vi "test - #98.vi"(8 "error in (no error)":errorcluster, 11 "TestCase in":refnum<class "testcase-Supported-Datatype.lvclass">) -> (0 "error out":errorcluster, 3 "TestCase out":refnum<class "testcase-Supported-Datatype.lvclass">)   [LabVIEW 2017, in "testcase-Supported-Datatype.lvclass"]
uses:
  testcase-Supported-Datatype.lvclass
  fb94dfaf-6f85-427f-a0fa-1e7f335e48cb.vi
  e57ab7a4-7139-4cc0-9c10-fbc2ee1cf7e2.vi
  addons/API-String-Arugments-Support/_Support/Data To API String Arguments.vi
  addons/API-String-Arugments-Support/_Support/Convert API String Arguments to Data(variant).vi
  <vilib>/addons/_JKI Toolkits/VI Tester/TestCase.llb/TestCase.lvclass
  C:/Program Files (x86)/National Instruments/LabVIEW 2017/vi.lib/addons/_JKI Toolkits/VI Tester/TestCase.llb/TestCase.lvclass
panel:
  out "String 2":string
  out "Stimulus 3":T1={"Stimulus Type"=enum."Frequency Stepped Sweep", "Custom Stimulus Name"="", "Apply EQ"=FALSE, "Advanced View"=FALSE, "Sampling Rate"="Device Default", "Output Path"={"Output Path"="", "Sampling Rate"=48000}, "Frequency Stepped Sweep"={"Level"=0.35, "Unit"=0, "Resolution"=1, "Start (Hz)"=10000.0, "Stop (Hz)"=100.0, "Min cycles (#)"=10.0, "Min Duration (s)"=0.01, "Steps (#)"=0}, "Frequency Log Sweep"={"Level"=0.35, "Unit"=0, "Start (Hz)"=100.0, "Stop (Hz)"=10000.0, "Sweep Time (s)"=2.0}, "Log Amplitude Sweep"={"Freq"=1000.0, "Steps (#)"=20.0, "Start"=1.0, "Unit"=0, "Cycles （#)"=10.0, "Stop"=2.0}, "WAV"={"Level"=0.35, "Unit"=0, "WAV File Path"=path "", "WAV File Channel"=0}, "Noise"={"Level"=0.35, "Unit"=0, "Noise Type"=enum."Pink Noise", "Min (Hz)"=100.0, "Max (Hz)"=20000.0, "Duration (s)"=2.0}, "Multitone"={"Level"=0.35, "Unit"=0, "Resolution"=1, "Min (Hz)"=100.0, "Max (Hz)"=10000.0, "Duration (s)"=2.0, "Tones (#)"=10}, "Stimulus List"=[]} {"Multitone"."Duration (s)" format="%#_6p"; "Multitone"."Max (Hz)" format="%#_6p"; "Multitone"."Min (Hz)" format="%#_6p"; "Multitone"."Resolution" items=["R10 (1/3 Oct.)", "R20 (1/6 Oct.)", "R40 (1/12 Oct.)", "R80 (1/24 Oct.)", "User Def. Log", "User Def. Lin"]; "Multitone"."Unit" items=["V RMS"]; "Multitone"."Level" format="%#_6p"; "Noise"."Max (Hz)" format="%#_6p"; "Noise"."Min (Hz)" format="%#_6p"; "Noise"."Unit" items=["V RMS"]; "Noise"."Level" format="%#_6p"; "WAV"."WAV File Channel" items=["Mono"]; "WAV"."Unit" items=["V RMS"]; "WAV"."Level" format="%#_6p"; "Log Amplitude Sweep"."Stop" format="%#_6p"; "Log Amplitude Sweep"."Cycles （#)" format="%#_6p"; "Log Amplitude Sweep"."Unit" items=["V RMS"]; "Log Amplitude Sweep"."Start" format="%#_6p"; "Log Amplitude Sweep"."Steps (#)" format="%#_6p"; "Log Amplitude Sweep"."Freq" format="%#_6p"; "Frequency Log Sweep"."Sweep Time (s)" format="%#_6p"; "Frequency Log Sweep"."Stop (Hz)" format="%#_6p"; "Frequency Log Sweep"."Start (Hz)" format="%#_6p"; "Frequency Log Sweep"."Unit" items=["V RMS"]; "Frequency Log Sweep"."Level" format="%#_6p"; "Frequency Stepped Sweep"."Min Duration (s)" format="%#_6p"; "Frequency Stepped Sweep"."Min cycles (#)" format="%#_6p"; "Frequency Stepped Sweep"."Stop (Hz)" format="%#_6p"; "Frequency Stepped Sweep"."Start (Hz)" format="%#_6p"; "Frequency Stepped Sweep"."Resolution" items=["R10 (1/3 Oct.)", "R20 (1/6 Oct.)", "R40 (1/12 Oct.)", "R80 (1/24 Oct.)", "User Def. Log", "User Def. Lin"]; "Frequency Stepped Sweep"."Unit" items=["V RMS"]; "Frequency Stepped Sweep"."Level" format="%#_6p"}
  in  "Stimulus 4":T1={"Stimulus Type"=enum."Frequency Log Sweep", "Custom Stimulus Name"="20-10k Chirp", "Apply EQ"=FALSE, "Advanced View"=TRUE, "Sampling Rate"="Device Default", "Output Path"={"Output Path"="Output 1", "Sampling Rate"=44100}, "Frequency Stepped Sweep"={"Level"=0.25, "Unit"=0, "Resolution"=0, "Start (Hz)"=100.0, "Stop (Hz)"=20000.0, "Min cycles (#)"=10.0, "Min Duration (s)"=0.01, "Steps (#)"=24}, "Frequency Log Sweep"={"Level"=0.25, "Unit"=0, "Start (Hz)"=20.0, "Stop (Hz)"=10000.0, "Sweep Time (s)"=1.0}, "Log Amplitude Sweep"={"Freq"=0.0, "Steps (#)"=0.0, "Start"=0.0, "Unit"=0, "Cycles （#)"=0.0, "Stop"=0.0}, "WAV"={"Level"=0.35000000000000003, "Unit"=0, "WAV File Path"=path "", "WAV File Channel"=0}, "Noise"={"Level"=0.35000000000000003, "Unit"=0, "Noise Type"=enum."Pink Noise", "Min (Hz)"=0.0, "Max (Hz)"=0.0, "Duration (s)"=0.0}, "Multitone"={"Level"=0.35000000000000003, "Unit"=0, "Resolution"=0, "Min (Hz)"=0.0, "Max (Hz)"=0.0, "Duration (s)"=0.0, "Tones (#)"=0}, "Stimulus List"=[["Frequency Stepped Sweep", "No", "0.588187", "33"]]} {"Multitone"."Duration (s)" format="%#_6p"; "Multitone"."Max (Hz)" format="%#_6p"; "Multitone"."Min (Hz)" format="%#_6p"; "Multitone"."Resolution" items=["R10 (1/3 Oct.)", "R20 (1/6 Oct.)", "R40 (1/12 Oct.)", "R80 (1/24 Oct.)", "User Def. Log", "User Def. Lin"]; "Multitone"."Unit" items=["V RMS"]; "Multitone"."Level" format="%#_6p"; "Noise"."Max (Hz)" format="%#_6p"; "Noise"."Min (Hz)" format="%#_6p"; "Noise"."Unit" items=["V RMS"]; "Noise"."Level" format="%#_6p"; "WAV"."WAV File Channel" items=["Mono"]; "WAV"."Unit" items=["V RMS"]; "WAV"."Level" format="%#_6p"; "Log Amplitude Sweep"."Stop" format="%#_6p"; "Log Amplitude Sweep"."Cycles （#)" format="%#_6p"; "Log Amplitude Sweep"."Unit" items=["V RMS"]; "Log Amplitude Sweep"."Start" format="%#_6p"; "Log Amplitude Sweep"."Steps (#)" format="%#_6p"; "Log Amplitude Sweep"."Freq" format="%#_6p"; "Frequency Log Sweep"."Sweep Time (s)" format="%#_6p"; "Frequency Log Sweep"."Stop (Hz)" format="%#_6p"; "Frequency Log Sweep"."Start (Hz)" format="%#_6p"; "Frequency Log Sweep"."Unit" items=["V RMS"]; "Frequency Log Sweep"."Level" format="%#_6p"; "Frequency Stepped Sweep"."Min Duration (s)" format="%#_6p"; "Frequency Stepped Sweep"."Min cycles (#)" format="%#_6p"; "Frequency Stepped Sweep"."Stop (Hz)" format="%#_6p"; "Frequency Stepped Sweep"."Start (Hz)" format="%#_6p"; "Frequency Stepped Sweep"."Resolution" items=["R10 (1/3 Oct.)", "R20 (1/6 Oct.)", "R40 (1/12 Oct.)", "R80 (1/24 Oct.)", "User Def. Log", "User Def. Lin"]; "Frequency Stepped Sweep"."Unit" items=["V RMS"]; "Frequency Stepped Sweep"."Level" format="%#_6p"}
  # "HERE"
  # "Hz"
  # "Hz"
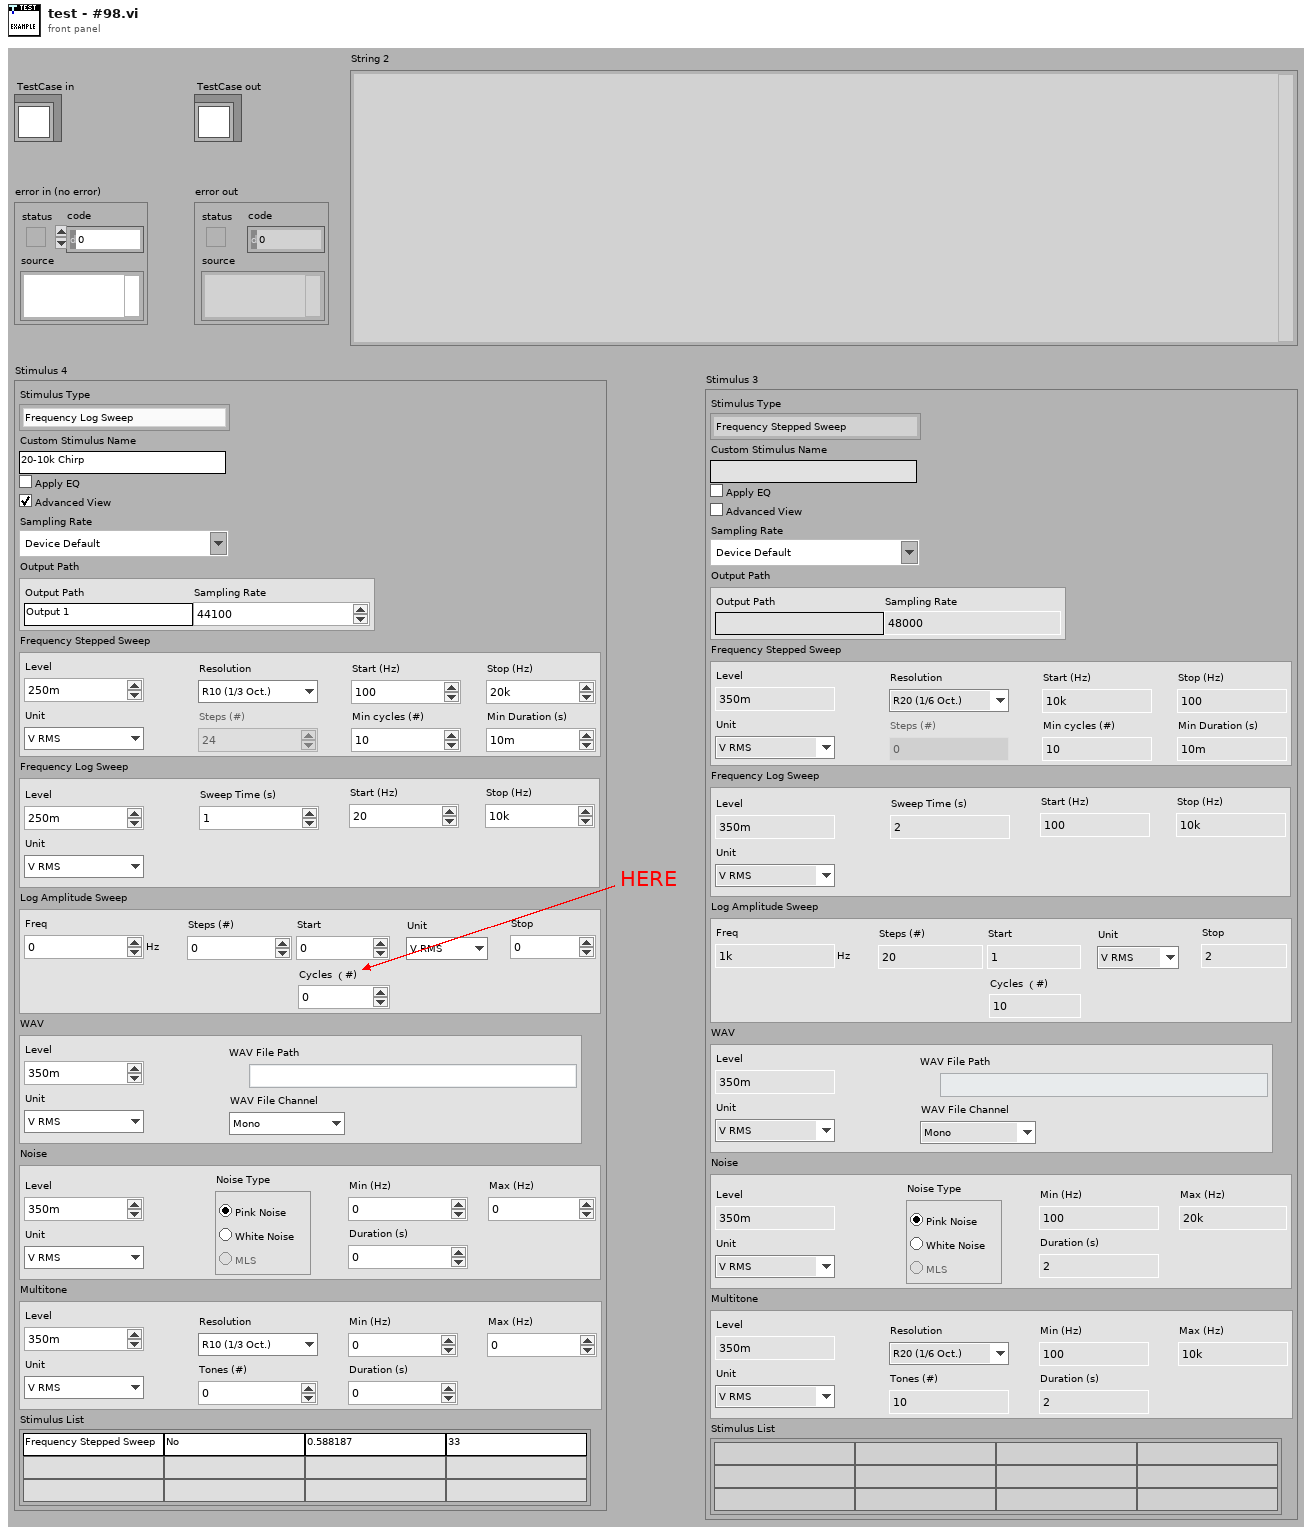
[diagram p1: front panel]
types:
  T1 = cluster{"Stimulus Type":enum32{"Frequency Stepped Sweep", "Frequency Log Sweep", "Log Amplitude Sweep", "WAV", "Noise", "Multitone"}, "Custom Stimulus Name":string, "Apply EQ":bool, "Advanced View":bool, "Sampling Rate":string, "Output Path":cluster{"Output Path":string, "Sampling Rate":i32}, "Frequency Stepped Sweep":cluster{"Level":dbl, "Unit":u16, "Resolution":u16, "Start (Hz)":dbl, "Stop (Hz)":dbl, "Min cycles (#)":dbl, "Min Duration (s)":dbl, "Steps (#)":i32}, "Frequency Log Sweep":cluster{"Level":dbl, "Unit":u16, "Start (Hz)":dbl, "Stop (Hz)":dbl, "Sweep Time (s)":dbl}, "Log Amplitude Sweep":cluster{"Freq":dbl, "Steps (#)":dbl, "Start":dbl, "Unit":u16, "Cycles （#)":dbl, "Stop":dbl}, "WAV":cluster{"Level":dbl, "Unit":u16, "WAV File Path":path, "WAV File Channel":u16}, "Noise":cluster{"Level":dbl, "Unit":u16, "Noise Type":enum32{"Pink Noise", "White Noise", "MLS"}, "Min (Hz)":dbl, "Max (Hz)":dbl, "Duration (s)":dbl}, "Multitone":cluster{"Level":dbl, "Unit":u16, "Resolution":u16, "Min (Hz)":dbl, "Max (Hz)":dbl, "Duration (s)":dbl, "Tones (#)":i32}, "Stimulus List":string[][]}
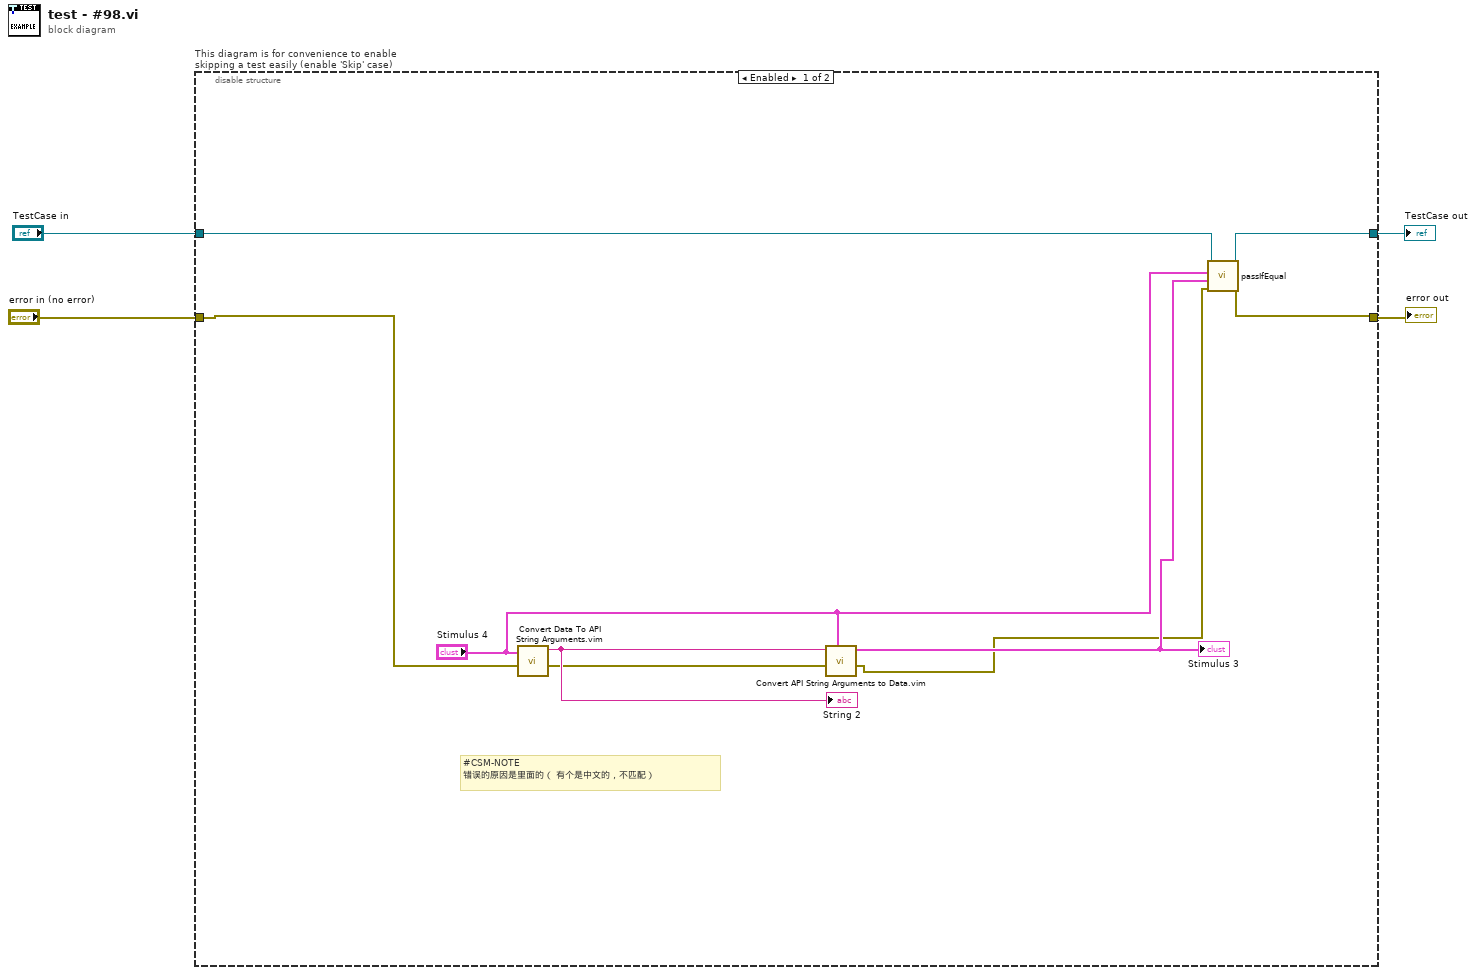
[diagram p0: block diagram]
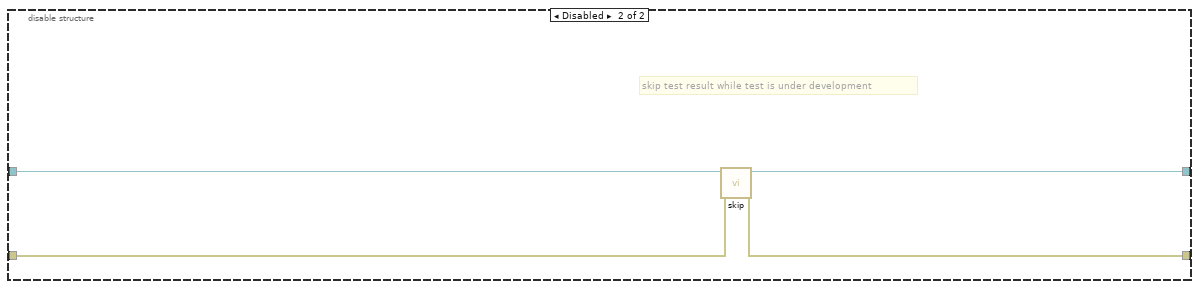
[diagram p2: hidden frame]
diagram:
  n1 = disable-structure "This diagram is for convenience to enable skipping a test easily (enable 'Skip' case)" shown="Enabled" {
    disable-tunnel: "TestCase in" -> [w13 w17]
    disable-tunnel: [w12 w15] -> w1
    disable-tunnel: [w11 w16] -> w3
    disable-tunnel: "error in (no error)" -> [w7 w14]
    frame Enabled {
      # "#CSM-NOTE\n错误的原因是里面的（ 有个是中文的，不匹配）"
      n2 = call "Convert Data To API String Arguments.vim"("error in (no error)"=w7, "Data"="Stimulus 4") -> ("error out"=w6:errorcluster, "API String"=w10:string)  [unwired: 6 in]
      "String 2" <- w10
      n3 = call "Convert API String Arguments to Data.vim"("Reference Type"="Stimulus 4", "error in (no error)"=w6, "API String"=w10) -> ("error out"=w5:errorcluster, "Data"=w8:T1)  [unwired: 5 in]
      "Stimulus 3" <- w8
      n4 = call-dynamic "passIfEqual.vi"("error in (no error)"=w5, "y"=w8, "x"="Stimulus 4", "TestCase in"=w13) -> ("error out"=w11:errorcluster, "TestCase out"=w12:refnum<class "testcase-Supported-Datatype.lvclass">)  [unwired: 6 in]
    }
    frame Disabled {
      # "skip test result while test is under development"
      n5 = call <vilib>:"skip.vi"("error in (no error)"=w14, "TestCase in"=w17) -> ("error out"=w16:errorcluster, "TestCase out"=w15:refnum<class "testcase-Supported-Datatype.lvclass">)  [unwired: 8 in]
    }
  }
  "error out" <- w3
  "TestCase out" <- w1
